vi "getEvaluation.vi"(8 "error in (no error)":errorcluster, 11 "MultiTreeNode in":refnum<class "MultiTreeNode.lvclass">) -> (0 "error out":errorcluster, 2 "evaluation":cluster{"F":dbl, "G":dbl, "H":dbl}, 3 "MultiTreeNode out":refnum<class "MultiTreeNode.lvclass">)   [LabVIEW 2014, in "MultiTree.lvlib" / "MultiTreeNode.lvclass"]
uses:
  <userlib>/AdvancedDataStructures/ClassBased/MultiTreeNode/MultiTreeNode.lvclass
  <userlib>/AdvancedDataStructures/ClassBased/MultiTreeNode/MultiTreeNode.lvclass/MultiTreeNode.ctl
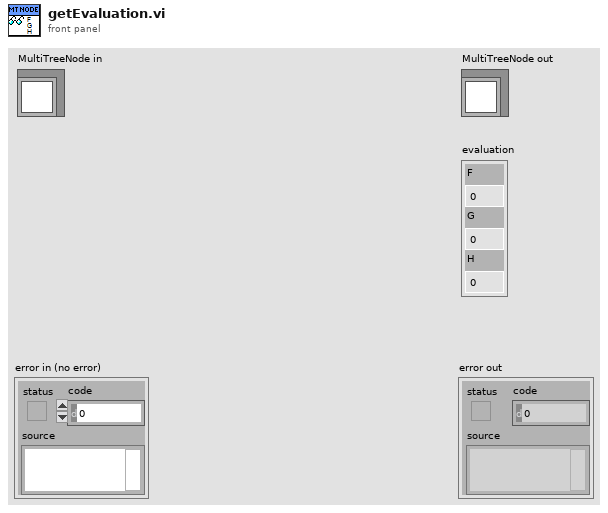
[diagram p1: front panel]
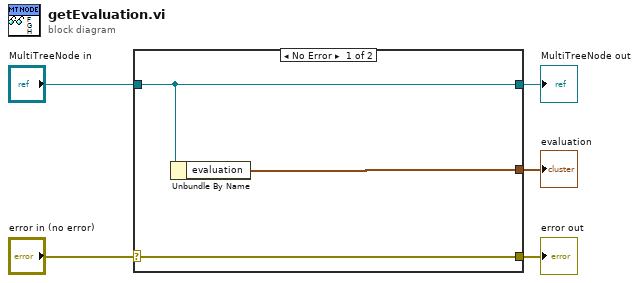
[diagram p0: block diagram]
diagram:
  n1 = case shown="No Error" "error in (no error)" {
    selector: "error in (no error)" -> [w8 w9]
    tunnel: [w8 w9] -> w4
    tunnel: [w7 w10] -> w2
    tunnel: "MultiTreeNode in" -> [w7 w10]
    tunnel: [w6 _] -> w1
    frame No Error {
      n2 = Unbundle By Name(w7) -> ("evaluation"=w6:cluster{"F":dbl, "G":dbl, "H":dbl})
    }
    frame Error {
    }
  }
  "error out" <- w4
  "MultiTreeNode out" <- w2
  "evaluation" <- w1
